vi "launch process ref bag -- V2.vi"(6 "launch item":T1, 7 "bag action":T2, 11 "process ref IN":refnum<vi>) -> (0 "values OUT":refnum<vi>[](array[refnum]), 1 "Keys OUT":T1[](array[typedef]), 3 "process ref OUT":refnum<vi>)   [LabVIEW 2020]
uses:
  launch items list.ctl
  que event bag action.ctl
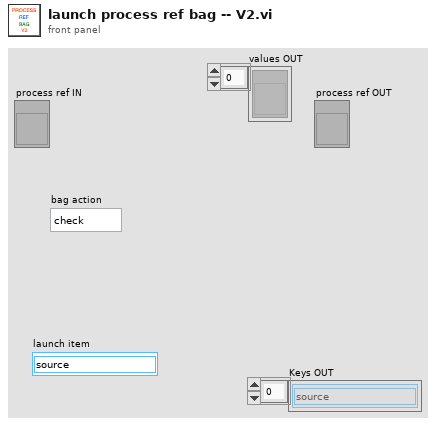
[diagram p1: front panel]
types:
  T1 = typedef "launch items list.ctl" = enum16{"source", "pll engine", "pll monitor", "sweeper engine", "sweeper monitor", "fitter"}
  T2 = typedef "que event bag action.ctl" = enum16{"check", "add", "init", "keys", "values"}
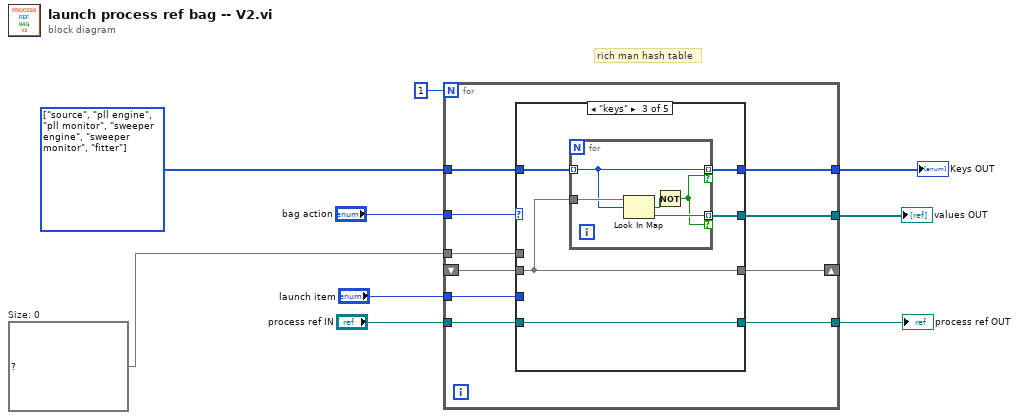
[diagram p0: block diagram]
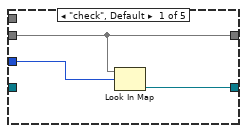
[diagram p2: hidden frame]
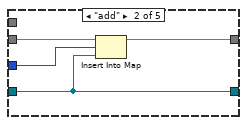
[diagram p3: hidden frame]
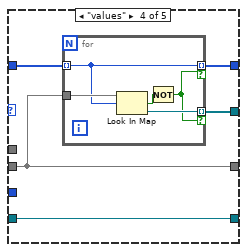
[diagram p4: hidden frame]
diagram:
  w3 = map{T1, refnum<vi>} {}  # Size: 0
  w6 = T1[] [enum."source", enum."pll engine", enum."pll monitor", enum."sweeper engine", enum."sweeper monitor", enum."fitter"] items=["source", "pll engine", "pll monitor", "sweeper engine", "sweeper monitor", "fitter"]
  # "rich man hash table"
  n1 = for {
    N: 1 -> [_]
    shift-right: [w14] -> _
    shift-left: _ -> [w19]
    tunnel: "bag action" -> [w18]
    tunnel: "launch item" -> [w17]
    tunnel: "process ref IN" -> [w16]
    tunnel: w3 -> [w15]
    tunnel: w6 -> [w13]
    tunnel: [w12] -> w1
    tunnel: [w11] -> w5
    tunnel: [w10] -> w2
    n2 = case shown="\"keys\"" w18 {
      tunnel: [w21 w26 w30 w40 w47] -> w14
      tunnel: w19 -> [w21 w23 w30 w40 _]
      tunnel: w17 -> [w22 w25 _ _ _]
      tunnel: w16 -> [_ w24 w31 w41 w48]
      tunnel: [w20 w24 w31 w41 w48] -> w10
      tunnel: w15 -> [_ _ _ _ w47]
      tunnel: w13 -> [_ _ w29 w39 _]
      tunnel: [_ _ w28 w38 _] -> w12
      tunnel: [_ _ w27 w37 _] -> w11
      frame "check", Default {
        n3 = Look In Map(map=w21, key=w22) -> (value=w20:refnum<vi>)  [unwired: 1 in, 1 out]
      }
      frame "add" {
        n4 = Insert Into Map(map in=w23, key=w25, value=w24) -> (map out=w26:map{T1, refnum<vi>})  [unwired: 2 out]
      }
      frame "keys" {
        n5 = for {
          tunnel: w30 -> [w36]
          tunnel: w29 -> [w33] mode=indexing
          tunnel: [w35] -> w28 mode=indexing if=w32
          tunnel: [w33] -> w27 mode=indexing if=w32
          n6 = Look In Map(map=w36, key=w33) -> (key not found?=w34:bool, value=w35:refnum<vi>)  [unwired: 1 in]
          n7 = Not(x=w34) -> (.not. x?=w32:bool)
        }
      }
      frame "values" {
        n8 = for {
          tunnel: w40 -> [w46]
          tunnel: w39 -> [w43] mode=indexing
          tunnel: [w45] -> w38 mode=indexing if=w42
          tunnel: [w43] -> w37 mode=indexing if=w42
          n9 = Look In Map(map=w46, key=w43) -> (key not found?=w44:bool, value=w45:refnum<vi>)  [unwired: 1 in]
          n10 = Not(x=w44) -> (.not. x?=w42:bool)
        }
      }
      frame "init" {
      }
    }
  }
  "process ref OUT" <- w2
  "Keys OUT" <- w5
  "values OUT" <- w1
